vi "Update Enable.vi"(8 "error in (no error)":errorcluster, 10 "Station Status":map{string, bool}(c390), 11 "Update station status in":refnum<class "Station Status.lvclass">) -> (0 "error out":errorcluster, 3 "Update station status out":refnum<class "Station Status.lvclass">)   [LabVIEW 2021, in "Station State.lvlib" / "Station Status.lvclass"]
uses:
  Station Status.lvclass
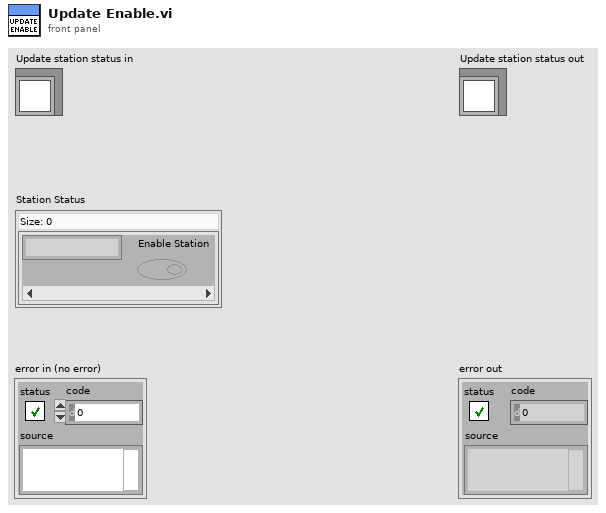
[diagram p1: front panel]
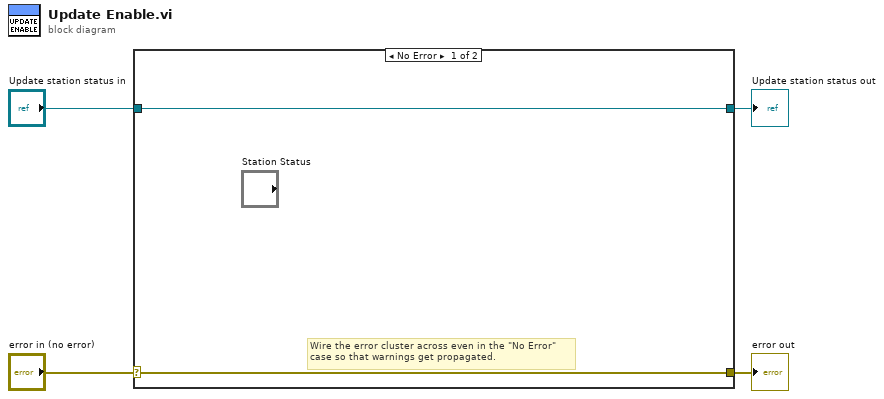
[diagram p0: block diagram]
diagram:
  n1 = case shown="No Error" "error in (no error)" {
    selector: "error in (no error)" -> [w5 w8]
    tunnel: [w5 w8] -> w3
    tunnel: [w6 w7] -> w1
    tunnel: "Update station status in" -> [w6 w7]
    frame No Error {
      # "Wire the error cluster across even in the \"No Error\"\ncase so that warnings get propagated."
    }
    frame Error {
    }
  }
  "error out" <- w3
  "Update station status out" <- w1
